vi "OKN model.vi"() -> ()   [LabVIEW 2013]
uses:
  biCNN/Cerebellum/Cerebellum.lvclass
  <vilib>/measure/NI_MABase.lvlib
panel:
  out "Retinal slip":dbl(graph)=4056.2226945124057
  out "Eye Vel 2":dbl[][](graph)
  out "Eye Vel":dbl[][](graph)
  out "Left Hemis":path
  out "Right Hemis":path
  out "preview 2":string
  out "preview":string
  in  "AERs for RIGHT":i32(listbox)
  in  "Existing Grids in Results/ 2":i32(listbox)
  in  "run":bool
  in  "AERs for LEFT":i32(listbox)
  in  "Existing Grids in Results/":i32(listbox)
  in  "Stim?":bool=TRUE
  out "Cycles":i32
  in  "stop":bool
  # "OKN System Simulation"
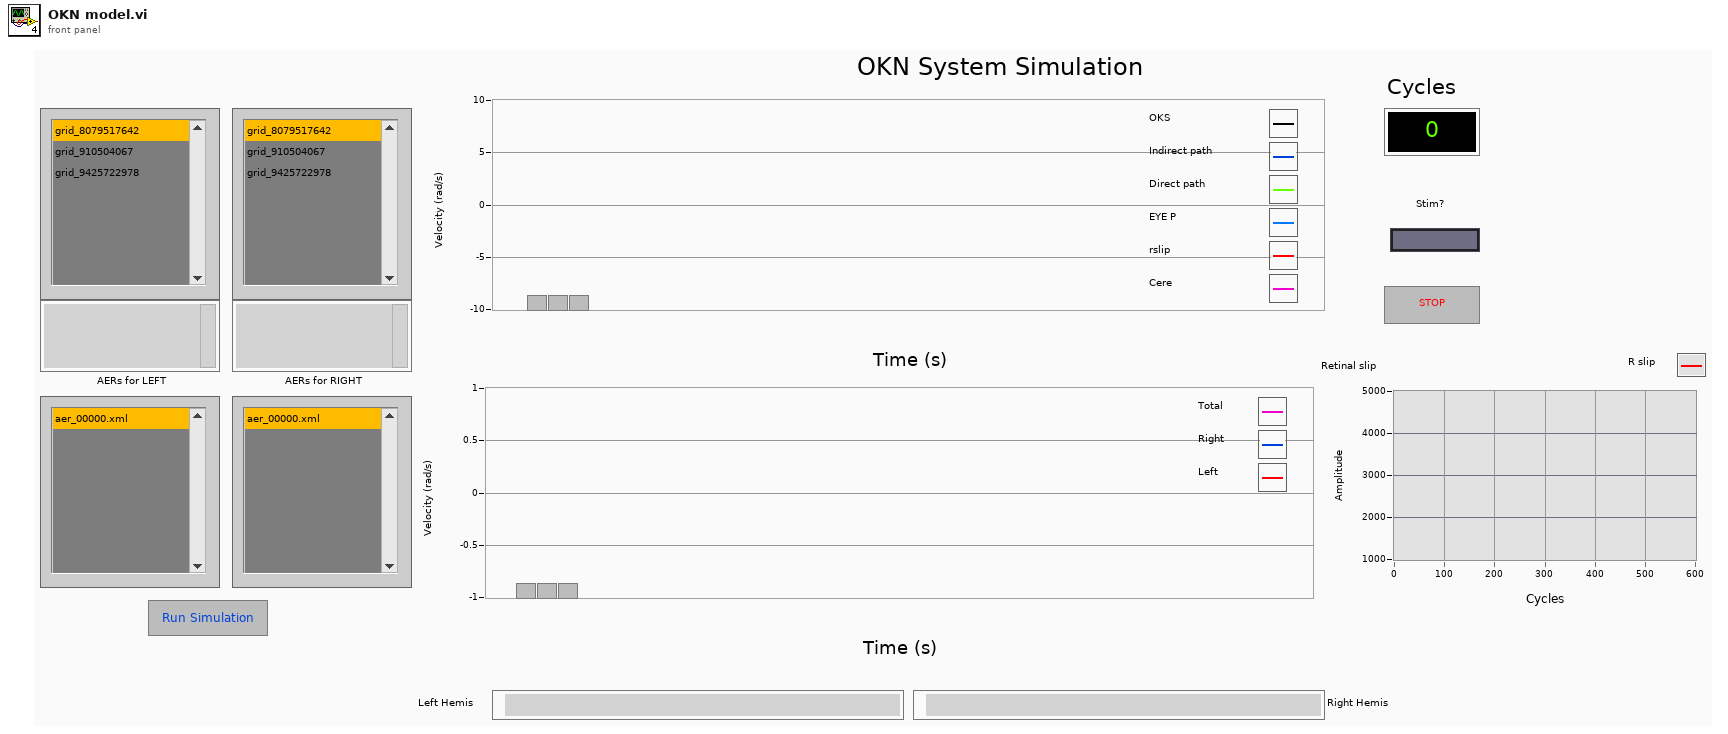
[diagram p1: front panel]
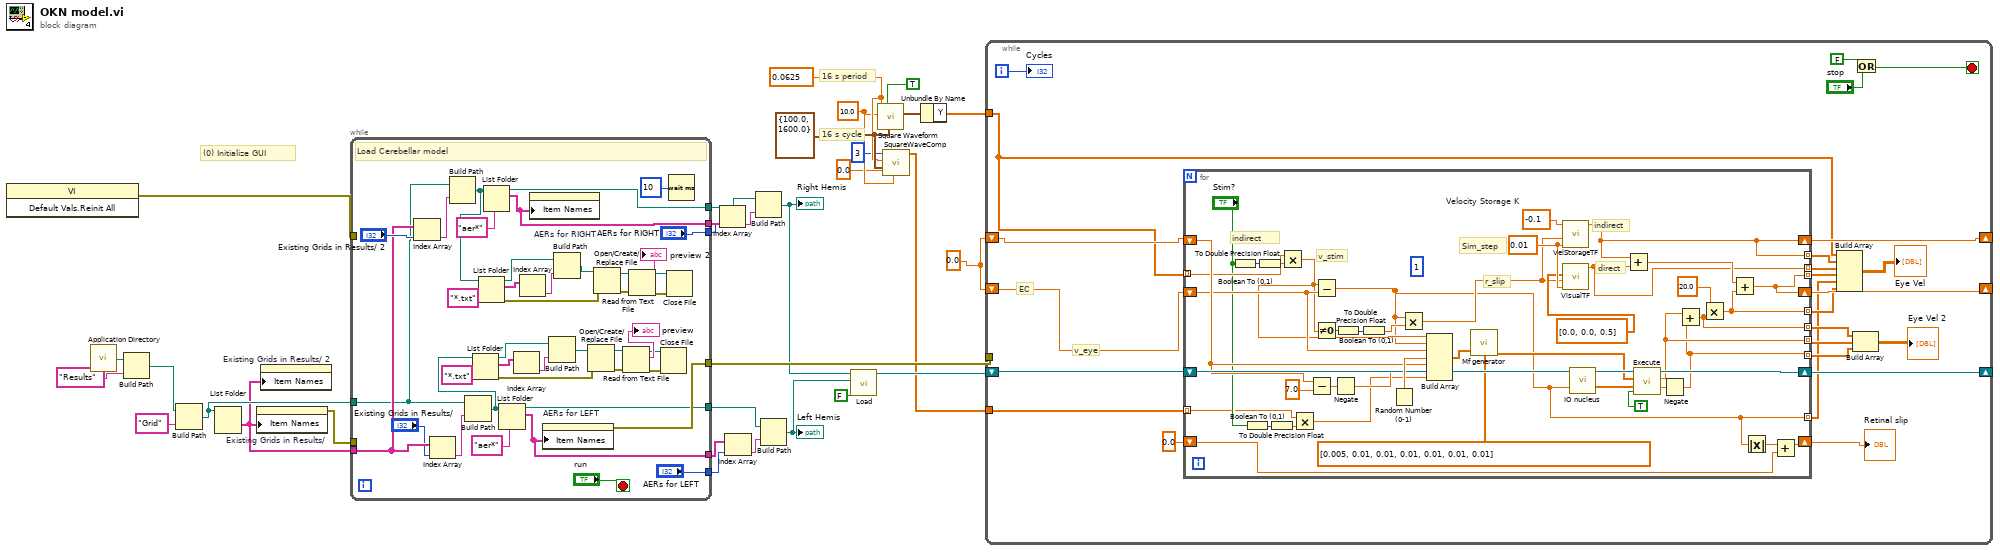
[diagram p0: block diagram]
diagram:
  w5 = 0.0625 ("frequency")
  w6 = cluster{"Fs":dbl, "#s":dbl} {"Fs"=100.0, "#s"=1600.0} ("sampling info")
  w2 = 10.0 ("offset")
  w7 = 0.0 ("NonDelayed Output")
  # "16 s period"
  # "16 s cycle"
  # "(0) Initialize GUI"
  n1 = invoke class="VI" method="Default Vals.Reinit All"() -> (error out=w22:errorcluster)  [unwired: 3 in, 2 out]
  n2 = call <vilib>:"Application Directory.vi"() -> ("Application Directory"=w30:path)
  n3 = Build Path(base path=w30, name or relative path="Results") -> (appended path=w28:path)
  n4 = Build Path(base path=w28, name or relative path="Grid") -> (appended path=w26:path)
  n5 = List Folder(path=w26) -> (folder names=w23:string[])  [unwired: 3 in, 3 out]
  n6 = property on="Existing Grids in Results/" class="LstBox (strict)"("Item Names"=w23) -> (error out=w27:errorcluster)  [unwired: 2 in, 1 out]
  n7 = property on="Existing Grids in Results/ 2" class="LstBox (strict)"("Item Names"=w23) -> ()  [unwired: 2 in, 2 out]
  n8 = while {
    tunnel: w27 -> [_]
    tunnel: w23 -> [w66]
    tunnel: w26 -> [w64]
    tunnel: [w70] -> w25
    tunnel: [w69] -> w16
    tunnel: w22 -> [_]
    tunnel: [w37] -> w17
    tunnel: [w36] -> w21
    tunnel: [w35] -> w19
    tunnel: ["AERs for LEFT"] -> w12
    tunnel: ["AERs for RIGHT"] -> w11
    stop <- "run" stop-if-true
    # "Load Cerebellar model"
    n9 = Index Array(array=w66, index="Existing Grids in Results/ 2") -> (element=w65:string)
    n10 = Index Array(array=w66, index="Existing Grids in Results/") -> (element=w72:string)
    n11 = Build Path(base path=w64, name or relative path=w65) -> (appended path=w56:path)
    n12 = Build Path(base path=w64, name or relative path=w72) -> (appended path=w44:path)
    n13 = List Folder(path=w44, pattern="*.txt") -> (path out=w41:path, filenames=w49:string[], error out=w47:errorcluster)  [unwired: 2 in, 1 out]
    n14 = List Folder(path=w56, pattern="*.txt") -> (path out=w53:path, filenames=w54:string[], error out=w57:errorcluster)  [unwired: 2 in, 1 out]
    n15 = List Folder(path=w56, pattern="aer*") -> (path out=w35:path, filenames=w36:string[])  [unwired: 2 in, 2 out]
    n16 = List Folder(path=w44, pattern="aer*") -> (path out=w69:path, filenames=w37:string[])  [unwired: 2 in, 2 out]
    n17 = Index Array(array=w49) -> (element=w42:string)  [unwired: 1 in]
    n18 = Index Array(array=w54) -> (element=w52:string)  [unwired: 1 in]
    n19 = property on="AERs for RIGHT" class="LstBox (strict)"("Item Names"=w36) -> ()  [unwired: 2 in, 2 out]
    n20 = property on="AERs for LEFT" class="LstBox (strict)"("Item Names"=w37) -> (error out=w70:errorcluster)  [unwired: 2 in, 1 out]
    n21 = Build Path(base path=w41, name or relative path=w42) -> (appended path=w43:path)
    n22 = Build Path(base path=w53, name or relative path=w52) -> (appended path=w51:path)
    n23 = Open/Create/Replace File(file path (use dialog)=w43, error in=w47) -> (refnum out=w38:refnum<file>, error out=w45:errorcluster)  [unwired: 4 in, 1 out]
    n24 = Open/Create/Replace File(file path (use dialog)=w51, error in=w57) -> (refnum out=w62:refnum<file>, error out=w63:errorcluster)  [unwired: 4 in, 1 out]
    n25 = Read from Text File(file (use dialog)=w38, error in=w45) -> (refnum out=w39:refnum<file>, text=→"preview":string, error out=w46:errorcluster)  [unwired: 2 in, 1 out]
    n26 = Read from Text File(file (use dialog)=w62, error in=w63) -> (refnum out=w60:refnum<file>, text=→"preview 2":string, error out=w61:errorcluster)  [unwired: 2 in, 1 out]
    n27 = Close File(refnum=w39, error in=w46) -> ()  [unwired: 2 out]
    n28 = Close File(refnum=w60, error in=w61) -> ()  [unwired: 2 out]
    n29 = Wait (ms)(milliseconds to wait=u32 10) -> ()  [unwired: 1 out]
  }
  n30 = Index Array(array=w21, index=w11) -> (element=w20:string)
  n31 = Index Array(array=w17, index=w12) -> (element=w18:string)
  n32 = Build Path(base path=w19, name or relative path=w20) -> (appended path=w15:path)
  "Right Hemis" <- w15
  n33 = Build Path(base path=w16, name or relative path=w18) -> (appended path=w14:path)
  "Left Hemis" <- w14
  n34 = call "Load.vi"("Trained?"=FALSE, "Left Hem Path"=w14, "Right Hem Path"=w15) -> ("Cerebellum out"=w13:refnum<class "Cerebellum.lvclass">)  [unwired: 8 in]
  n35 = call <vilib>:"Square Waveform.vi"("sampling info"=w6, "reset signal"=TRUE, "amplitude"=w2, "frequency"=w5) -> ("signal out"=w10:waveform(dbl))  [unwired: 6 in, 1 out]
  n36 = call "SquareWaveComp.vi"("Amp"=w2, "Offset"=0.0, "sampling info"=w6, "frequency"=w5, "Components"=3) -> ("Decomposed"=w3:dbl[])  [unwired: 6 in]
  n37 = Unbundle By Name(w10) -> ("Y"=w8:dbl[])
  n38 = while {
    shift-right: [w91] -> _
    shift-left: w7 -> [w87]
    shift-right: [w92] -> _
    shift-left: w13 -> [w93]
    tunnel: w25 -> [_]
    tunnel: w8 -> [w81]
    shift-right: [w90] -> _
    shift-left: w7 -> [w89]
    tunnel: w3 -> [w75]
    i -> [w88]
    stop <- w95 stop-if-true
    # "EC"
    # "v_eye"
    n39 = for {
      shift-right: [w120] -> w91
      shift-left: w87 -> [w110]
      tunnel: w81 -> [w109] mode=indexing
      shift-right: [w133] -> w92
      shift-left: w93 -> [w134]
      shift-right: [w123] -> w90
      shift-left: w89 -> [w111]
      tunnel: [w97] -> w83 mode=indexing
      tunnel: [w124] -> w84 mode=indexing
      tunnel: [w123] -> w80 mode=indexing
      tunnel: [w122] -> w79 mode=indexing
      tunnel: [w121] -> w85 mode=indexing
      tunnel: [w120] -> w78 mode=indexing
      tunnel: [w117] -> w77 mode=indexing
      tunnel: [w99] -> w76 mode=indexing
      tunnel: w75 -> [w104] mode=indexing
      shift-right: [w102] -> w73
      shift-left: 0.0 -> [w101]
      (unwired) 1 ("FIFO size")
      w137 = 0.01
      w139 = -0.1  # Velocity Storage K
      # "indirect"
      # "r_slip"
      # "indirect"
      # "direct"
      # "Sim_step"
      # "v_stim"
      n40 = Boolean To (0,1)(Boolean="Stim?") -> (0, 1=w127:i16)
      n41 = Boolean To (0,1)(Boolean="Stim?") -> (0, 1=w106:i16)
      n42 = To Double Precision Float(number=w127) -> (double precision float=w125:dbl)
      n43 = To Double Precision Float(number=w106) -> (double precision float=w107:dbl)
      n44 = Multiply(x=w109, y=w125) -> (x*y=w108:dbl)
      n45 = Multiply(x=w104, y=w107) -> (x*y=w100:dbl)
      n46 = Subtract(x=w111, y=7.0) -> (x-y=w118:dbl)
      n47 = Subtract(x=w108, y=w110) -> (x-y=w99:dbl)
      n48 = Not Equal To 0?(x=w108) -> (x != 0?=w116:bool)
      n49 = Negate(x=w118) -> (-x=w113:dbl)
      n50 = Boolean To (0,1)(Boolean=w116) -> (0, 1=w115:i16)
      n51 = To Double Precision Float(number=w115) -> (double precision float=w114:dbl)
      n52 = Random Number (0-1)() -> (number: 0 to 1=w136:dbl)
      n53 = Multiply(x=w99, y=w114) -> (x*y=w112:dbl)
      n54 = Build Array(w108, w99, w110, w136, w111, w113, w100) -> (w138:dbl[])
      n55 = call "Mf generator.vi"("Inputs"=w138, "Gains"=dbl[] [0.005, 0.01, 0.01, 0.01, 0.01, 0.01, 0.01]) -> ("Mfs Inputs"=w132:dbl[])  [unwired: 1 in]
      n56 = call "VelStorageTF.vi"("Int. Step (ms)"=w137, "Retinal Slip"=w112, "Leak cnt"=w139) -> ("Eye position"=w123:dbl)  [unwired: 8 in]
      n57 = call "VisualTF.vi"("Int. Step (ms)"=w137, "Action u(t)"=w112, "State Space Coeff y(t)"=dbl[] [0.0, 0.0, 0.5]) -> ("NonDelayed Output"=w122:dbl)  [unwired: 8 in]
      n58 = call "IO nucleus.vi"("cf"=w99) -> ("cfs"=w128:dbl[])  [unwired: 2 in]
      n59 = Add(x=w123, y=w122) -> (x+y=w135:dbl)
      n60 = call "Execute.vi"("Active?"=TRUE, "cfs"=w128, "Inputs"=w132, "Cerebellum in"=w134) -> ("PC Left"=w98:dbl, "PC Right"=w124:dbl, "Cerebellum out"=w133:refnum<class "Cerebellum.lvclass">)  [unwired: 5 in]
      n61 = Negate(x=w98) -> (-x=w97:dbl)
      n62 = Add(x=w124, y=w97) -> (x+y=w121:dbl)
      n63 = Multiply(x=20.0, y=w121) -> (x*y=w117:dbl)
      n64 = Add(x=w135, y=w117) -> (x+y=w120:dbl)
      n65 = Absolute Value(x=w99) -> (abs(x)=w103:dbl)
      n66 = Add(x=w103, y=w101) -> (x+y=w102:dbl)
    }
    "Retinal slip" <- w73
    n67 = Build Array(w81, w80, w79, w78, w76, w77) -> (→"Eye Vel":dbl[][])
    n68 = Build Array(w85, w84, w83) -> (→"Eye Vel 2":dbl[][])
    n69 = Or(x=FALSE, y="stop") -> (x .or. y?=w95:bool)
    "Cycles" <- w88
  }
